vi "Omron Serial FINS-Write Data(I16 Element).vi"(8 "error in":errorcluster, 9 "Data":i16, 10 "Write Setting(I16 Element)":T1={"I/O Memory Address"=130, "Data Address"=0} {"I/O Memory Address" items=["DM"=130, "CIO"=176, "WR"=177, "HR"=178, "AR"=179, "TIM"=137, "EM"=152]}, 11 "Buffer Data In":T2={"VISA Resource Name"="", "Wait For Read(ms)"=50, "Command Code"=enum."Memory area read", "Command String"="", "Read Bytes"=0, "Response String"=""}) -> (0 "error out":errorcluster, 3 "Buffer Data Out":T2={"VISA Resource Name"="", "Wait For Read(ms)"=50, "Command Code"=enum."Memory area read", "Command String"="", "Read Bytes"=0, "Response String"=""})   [LabVIEW 2016]
uses:
  Data Def/Omron Serial FINS-Buffer Data.ctl
  Data Def/Omron Serial FINS-Command Code.ctl
  Data Def/Omron Serial FINS-FINS Command Frame.ctl
  Data Def/Omron Serial FINS-Memory Area Write Data.ctl
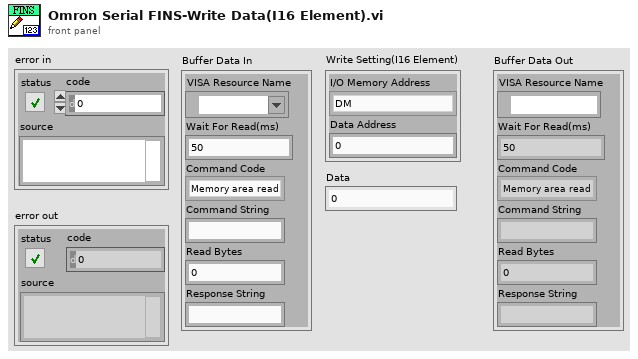
[diagram p1: front panel]
types:
  T1 = cluster{"I/O Memory Address":i32, "Data Address":u32}
  T2 = typedef "Omron Serial FINS-Buffer Data.ctl" = cluster{"VISA Resource Name":refnum<visa-resource-name>, "Wait For Read(ms)":u32, "Command Code":T3, "Command String":string, "Read Bytes":u32, "Response String":string}
  T3 = typedef "Omron Serial FINS-Command Code.ctl" = enum16{"Memory area read", "Memory area write"}
  T4 = typedef "Omron Serial FINS-Memory Area Write Data.ctl" = cluster{"I/O Memory Address":i32, "Beginning Address":u32, "No. Of Items":u32, "Data":i16[]}
  T5 = typedef "Omron Serial FINS-FINS Command Frame.ctl" = cluster{"Unit Number":u8, "Response Wait Time":u8, "Command Code":T3, "Command Data":variant}
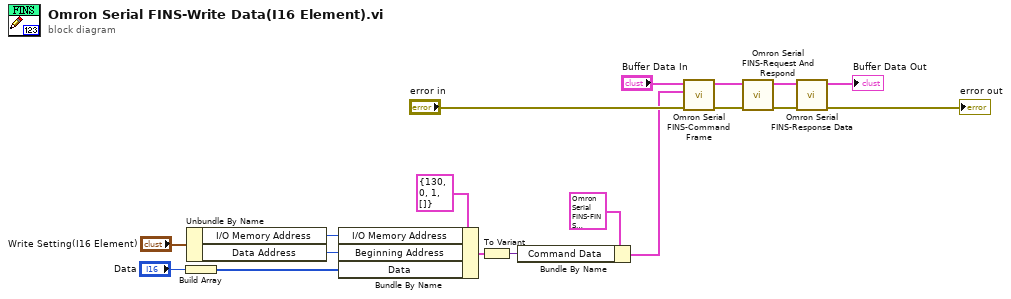
[diagram p0: block diagram]
diagram:
  n1 = Build Array("Data") -> (w1:i16[])
  n2 = Unbundle By Name("Write Setting(I16 Element)") -> ("I/O Memory Address"=w5:i32, "Data Address"=w4:u32)
  n3 = Bundle By Name(cluster=T4 {"I/O Memory Address"=130, "Beginning Address"=0, "No. Of Items"=1, "Data"=[]} ("Memory Area Write Data"), "I/O Memory Address"=w5, "Beginning Address"=w4, "Data"=w1) -> (w7:T4)
  n4 = To Variant(anything=w7) -> (Variant=w16:variant)
  n5 = Bundle By Name(cluster=T5 {"Unit Number"=0, "Response Wait Time"=0, "Command Code"=enum."Memory area write", "Command Data"=variant} ("FINS Command Frame"), "Command Data"=w16) -> (w14:T5)
  n6 = call "Omron Serial FINS-Command Frame.vi"("error in"="error in", "FINS Command Frame"=w14, "Buffer Data In"="Buffer Data In") -> ("error out"=w12:errorcluster, "Buffer Data Out"=w13:T2)  [unwired: 7 in]
  n7 = call "Omron Serial FINS-Request And Respond.vi"("error in"=w12, "Buffer Data In"=w13) -> ("error out"=w10:errorcluster, "Buffer Data Out"=w11:T2)  [unwired: 8 in]
  n8 = call "Omron Serial FINS-Response Data.vi"("error in"=w10, "Buffer Data In"=w11) -> ("error out"=→"error out":errorcluster, "Buffer Data Out"=→"Buffer Data Out":T2)  [unwired: 7 in, 1 out]
